vi "vipbBuild-nocli.vi"() -> (0 "error out":errorcluster)   [LabVIEW 2015]
uses:
  <vilib>/JKI/VIPM API/VIPM API_vipm_api.lvlib
panel:
  out "appended path":path
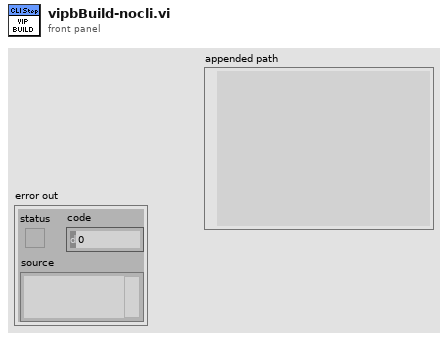
[diagram p1: front panel]
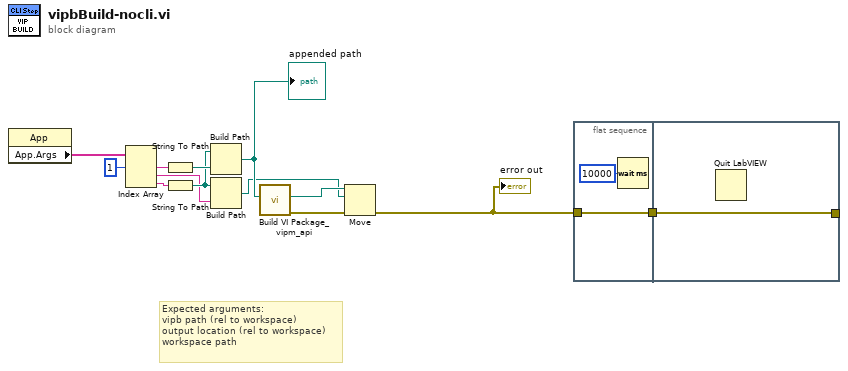
[diagram p0: block diagram]
diagram:
  # "Expected arguments:\nvipb path (rel to workspace)\noutput location (rel to workspace)\nworkspace path"
  n1 = property class="App"() -> ("App.Args"=w6:string[])  [unwired: 2 in, 2 out]
  n2 = Index Array(array=w6, index #1=1 ("index")) -> (element #1=w10:string, element #2=w7:string, element #3=w9:string)  [unwired: 2 in]
  n3 = String To Path(string=w10) -> (path=w13:path)
  n4 = String To Path(string=w9) -> (path=w8:path)
  n5 = Build Path(base path=w8, name or relative path=w13) -> (appended path=w11:path)
  "appended path" <- w11
  n6 = Build Path(base path=w8, name or relative path=w7) -> (appended path=w1:path)
  n7 = call <vilib>:"Build VI Package_vipm_api.vi"("Path to VIPB File"=w11) -> ("error out"=w12:errorcluster, "Build Output"=w2:path)  [unwired: 9 in]
  n8 = Move(source path=w2, error in=w12, 10:w1) -> (error out=w4:errorcluster)  [unwired: 2 in, 2 out]
  "error out" <- w4
  n9 = flat-sequence {
    tunnel: w4 -> [w15]
    tunnel: [w15] -> w3
    tunnel: [w16] -> _
    tunnel: w3 -> [w16]
    frame #0 {
      n10 = Wait (ms)(milliseconds to wait=u32 10000) -> ()  [unwired: 1 out]
    }
    frame #1 {
      n11 = Quit LabVIEW() -> ()  [unwired: 1 in]
    }
  }
